vi "Parse Path Array indexes.vi"(9 "error in (no error)":errorcluster, 11 "Path with leading Array element":string) -> (1 "error out":errorcluster, 2 "Indexes (empty means use all)":i32[](array[numeric]), 3 "Rest or Path":string, 4 "Max Index to parse":i32)   [LabVIEW 2024, in "JSONtext.lvlib"]
uses:
  JSONtext.lvlib
  Parsing State.ctl
  JSON Value Type.ctl
  Advance past Line Ending.vi
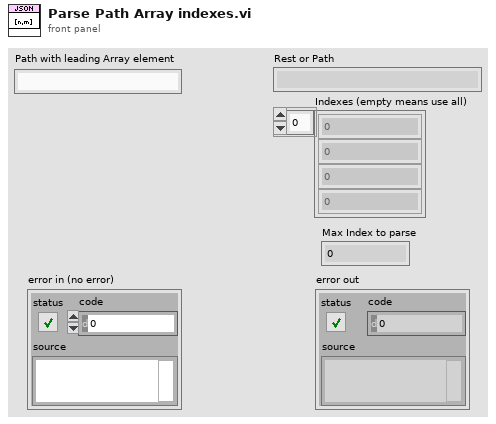
[diagram p1: front panel]
types:
  T1 = typedef "JSONtext.lvlib/Parsing State.ctl" = enum16{"Parser Error", "Object", "Array", "String", "Number/Other", "Leading Whitespace", "Object end", "Array end", "Value end"}
  T2 = typedef "JSONtext.lvlib/JSON Value Type.ctl" = enum16{"Not a JSON Value", "JSON Object", "JSON Array", "String", "Number", "true", "false", "null"}
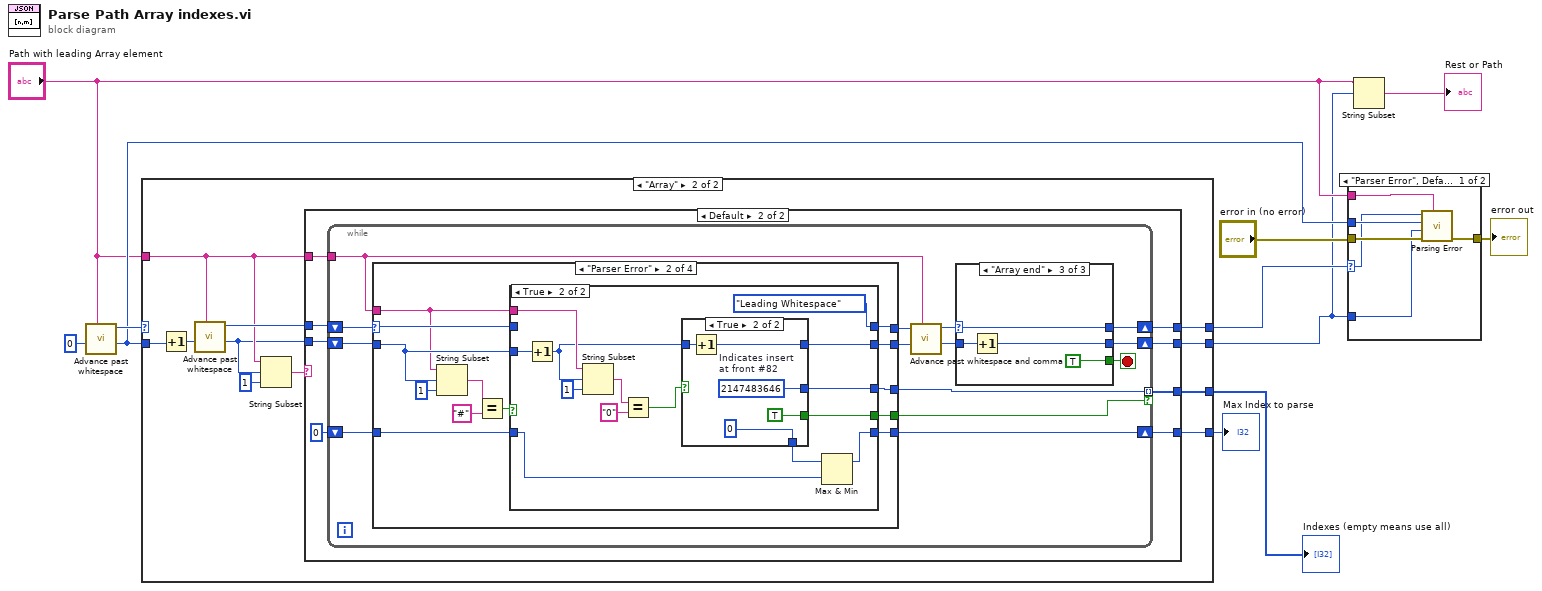
[diagram p0: block diagram]
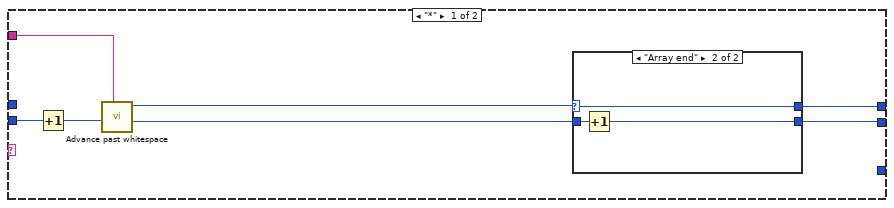
[diagram p3: hidden frame]
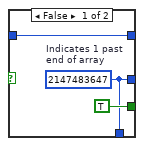
[diagram p7: hidden frame]
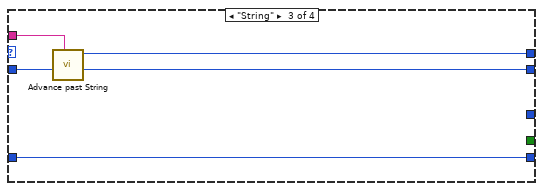
[diagram p8: hidden frame]
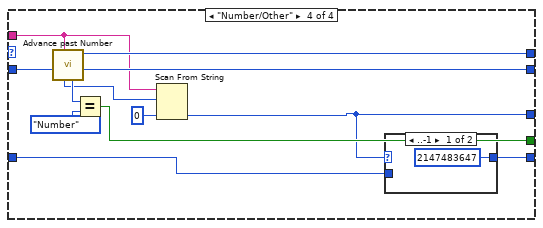
[diagram p9: hidden frame]
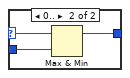
[diagram p10: hidden frame]
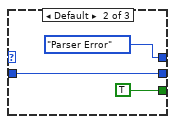
[diagram p12: hidden frame]
diagram:
  n1 = call "Advance past whitespace.vi"("JSON"="Path with leading Array element", "Offset"=0) -> ("Offset of first non-whitespace"=w7:i32, "Parser State"=w11:T1)  [unwired: 7 in, 1 out]
  n2 = case shown="\"Array\"" w11 {
    selector: w11 -> [w12 _]
    tunnel: w7 -> [w13 w24]
    tunnel: "Path with leading Array element" -> [_ w21]
    tunnel: [_ w17] -> w6
    tunnel: [w13 w16] -> w3
    tunnel: [w12 w15] -> w8
    tunnel: [_ w14] -> w1
    frame "Parser Error", Default {
    }
    frame "Array" {
      n3 = Increment(x=w24) -> (x+1=w22:i32)
      n4 = call "Advance past whitespace.vi"("JSON"=w21, "Offset"=w22) -> ("Offset of first non-whitespace"=w20:i32, "Parser State"=w23:T1)  [unwired: 7 in, 1 out]
      n5 = String Subset(string=w21, offset (0)=w20, length (rest)=1 ("length (rest)")) -> (substring=w18:string)
      n6 = case shown="Default" w18 {
        tunnel: w23 -> [_ w44]
        tunnel: w21 -> [w25 w43]
        tunnel: w20 -> [w31 w42]
        tunnel: [_ w41] -> w17
        tunnel: [w27 w40] -> w16
        tunnel: [w26 w39] -> w15
        tunnel: [_ w37] -> w14
        frame "*" {
          n7 = Increment(x=w31) -> (x+1=w30:i32)
          n8 = call "Advance past whitespace.vi"("JSON"=w25, "Offset"=w30) -> ("Offset of first non-whitespace"=w28:i32, "Parser State"=w29:T1)  [unwired: 7 in, 1 out]
          n9 = case shown="\"Array end\"" w29 {
            selector: w29 -> [w33 w34]
            tunnel: w28 -> [w32 w36]
            tunnel: [w32 w35] -> w27
            tunnel: [w33 w34] -> w26
            frame "Parser Error", Default {
            }
            frame "Array end" {
              n10 = Increment(x=w36) -> (x+1=w35:i32)
            }
          }
        }
        frame Default {
          n11 = while {
            tunnel: w43 -> [w51]
            shift-right: [w56] -> w40
            shift-left: w42 -> [w49]
            shift-right: [w52] -> w39
            shift-left: w44 -> [w50]
            tunnel: [w48] -> w41 mode=indexing if=w47
            shift-right: [w46] -> w37
            shift-left: 0 -> [w45]
            stop <- w55 stop-if-true
            n12 = case shown="\"Parser Error\"" w50 {
              selector: w50 -> [w61 w65 _ _]
              tunnel: w49 -> [w60 w67 w103 w114]
              tunnel: [w61 w68 w104 w116] -> w54
              tunnel: [w60 w66 w101 w115] -> w53
              tunnel: w51 -> [_ w62 w102 w110]
              tunnel: [_ w70 _ w107] -> w48
              tunnel: [_ w69 _ w111] -> w47
              tunnel: [w59 w64 w100 w106] -> w46
              tunnel: w45 -> [w59 w63 w100 w105]
              frame Default {
              }
              frame "Parser Error" {
                n13 = String Subset(string=w62, offset (0)=w67, length (rest)=1 ("length (rest)")) -> (substring=w73:string)
                n14 = Equal?(x=w73, y="#") -> (x = y?=w71:bool)
                n15 = case shown="True" w71 {
                  tunnel: [_ w89] -> w70
                  tunnel: [_ w91] -> w69
                  tunnel: [w77 Parsing_State."Leading Whitespace" ("Parser State")] -> w68
                  tunnel: w67 -> [w76 w85]
                  tunnel: [w76 w83] -> w66
                  tunnel: w65 -> [w77 _]
                  tunnel: [w75 w78] -> w64
                  tunnel: w63 -> [w75 w80]
                  tunnel: w62 -> [_ w82]
                  frame False {
                  }
                  frame True {
                    n16 = Increment(x=w85) -> (x+1=w81:i32)
                    n17 = String Subset(string=w82, offset (0)=w81, length (rest)=1 ("length (rest)")) -> (substring=w87:string)
                    n18 = Equal?(x=w87, y="0") -> (x = y?=w84:bool)
                    n19 = case shown="True" w84 {
                      tunnel: [TRUE TRUE] -> w91
                      tunnel: [w92 w98] -> w89
                      tunnel: w81 -> [w93 w97]
                      tunnel: [w93 w96] -> w83
                      tunnel: [w92 0 ("Indicates 1 past\nend of array")] -> w79
                      frame False {
                        w92 = 2147483647  # Indicates 1 past end of array
                      }
                      frame True {
                        w98 = 2147483646  # Indicates insert  at front #82
                        n20 = Increment(x=w97) -> (x+1=w96:i32)
                      }
                    }
                    n21 = Max & Min(x=w79, y=w80) -> (max(x,y)=w78:i32)  [unwired: 1 out]
                  }
                }
              }
              frame "String" {
                n22 = call "Advance past String.vi"("JSON"=w102, "Offset"=w103) -> ("Offset past match"=w101:i32, "State"=w104:T1)  [unwired: 7 in, 1 out]
              }
              frame "Number/Other" {
                n23 = call "Advance past Number.vi"("JSON"=w110, "Offset (0)"=w114) -> ("Offset past match"=w115:i32, "Parser State"=w116:T1, "JSON Value Type"=w113:T2, "Value start out"=w109:i32)  [unwired: 5 in, 1 out]
                n24 = Equal?(x=w113, y=JSON_Value_Type."Number") -> (x = y?=w111:bool)
                n25 = Scan From String(input string=w110, initial scan location=w109, default 1=0) -> (output 1=w107:i32)  [unwired: 2 in, 3 out]
                n26 = case shown="..-1" w107 {
                  selector: w107 -> [_ w120]
                  tunnel: [2147483647 w119] -> w106
                  tunnel: w105 -> [_ w118]
                  frame ..-1 {
                  }
                  frame 0.. {
                    n27 = Max & Min(x=w120, y=w118) -> (max(x,y)=w119:i32)  [unwired: 1 out]
                  }
                }
              }
            }
            n28 = call "Advance past whitespace and comma.vi"("JSON"=w51, "Offset"=w53, "State in"=w54) -> ("Offset past match"=w58:i32, "State"=w57:T1)  [unwired: 6 in, 1 out]
            n29 = case shown="\"Array end\"" w57 {
              selector: w57 -> [w121 _ w126]
              tunnel: [_ TRUE TRUE] -> w55
              tunnel: w58 -> [w122 w124 w128]
              tunnel: [w122 w124 w127] -> w56
              tunnel: [w121 Parsing_State."Parser Error" w126] -> w52
              frame "Number/Other" {
              }
              frame Default {
              }
              frame "Array end" {
                n30 = Increment(x=w128) -> (x+1=w127:i32)
              }
            }
          }
        }
      }
    }
  }
  "Indexes (empty means use all)" <- w6
  "Max Index to parse" <- w1
  n31 = case shown="\"Parser Error\", Default" w8 {
    selector: w8 -> [w130 _]
    tunnel: "Path with leading Array element" -> [w135 _]
    tunnel: "error in (no error)" -> [w134 w136]
    tunnel: [w133 w136] -> w9
    tunnel: w7 -> [w132 _]
    tunnel: w3 -> [w131 _]
    frame "Parser Error", Default {
      n32 = call "Parsing Error.vi"("JSON"=w135, "error in (no error)"=w134, "Offset past match"=w131, "Value start"=w132, "State"=w130) -> ("error out"=w133:errorcluster)  [unwired: 6 in]
    }
    frame "Array end" {
    }
  }
  "error out" <- w9
  n33 = String Subset(string="Path with leading Array element", offset (0)=w3) -> (substring=→"Rest or Path":string)  [unwired: 1 in]
